vi "Servicio to Hardware.vi"(8 "error in (no error)":errorcluster, 10 "Servicio seleccionado":string, 11 "UI in":refnum<class "UI.lvclass">) -> (0 "error out":errorcluster, 3 "UI out":refnum<class "UI.lvclass">)   [LabVIEW 2020, in "UI.lvlib" / "UI.lvclass"]
uses:
  UI.lvclass
  UI.lvclass/UI.ctl
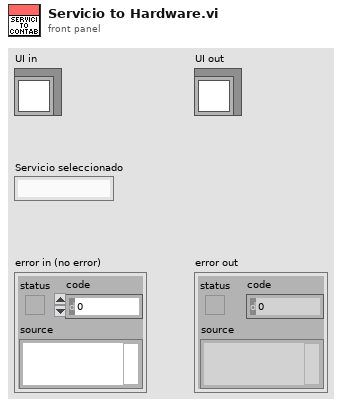
[diagram p1: front panel]
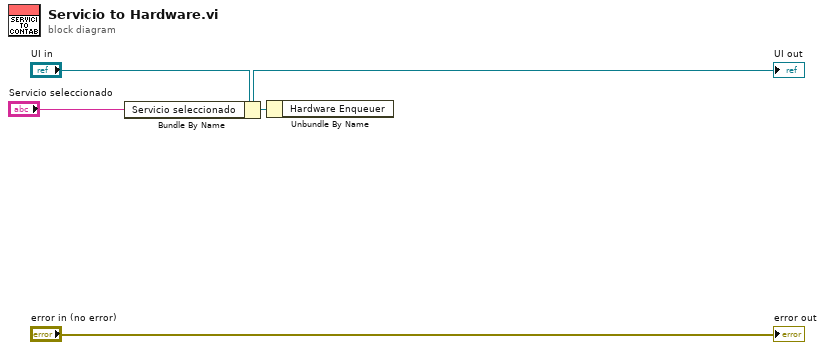
[diagram p0: block diagram]
diagram:
  n1 = Bundle By Name(cluster="UI in", "Servicio seleccionado"="Servicio seleccionado") -> (w1:refnum<class "UI.lvclass">)
  "UI out" <- w1
  n2 = Unbundle By Name(w1) -> ()  [unwired: 1 out]
  "error out" <- "error in (no error)"
